vi "1D Str to ITX Wave.vi"(1 "String":string[](array[string]), 2 "Wavename":string) -> (0 "ITX Wave":string)   [LabVIEW 2020, in "Data.ITX.lvclass"]
uses:
  Data.ITX.lvclass
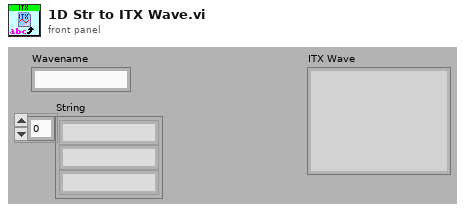
[diagram p1: front panel]
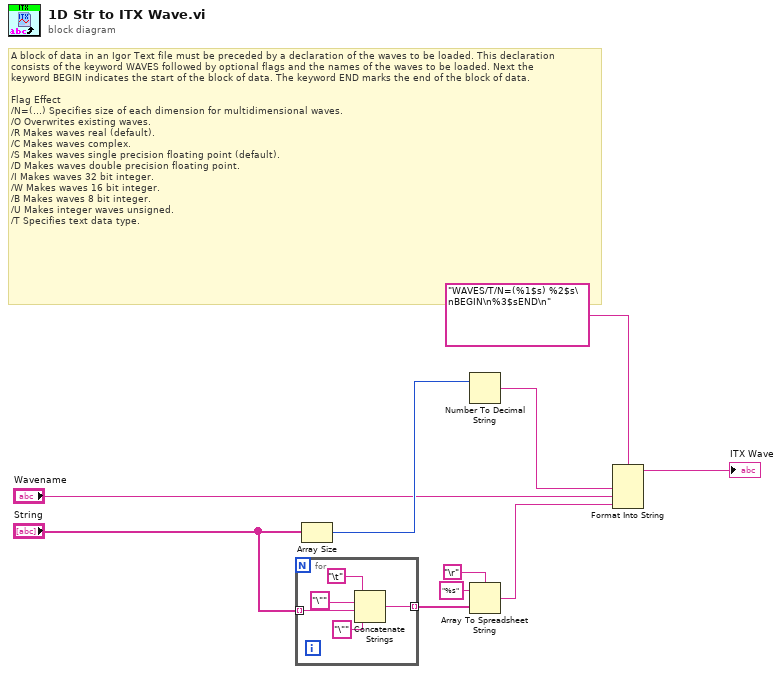
[diagram p0: block diagram]
diagram:
  # "A block of data in an Igor Text file must be preceded by a declaration of the waves to be loaded. This declaration\nconsists of the keyword WAVES followed by optional flags and the names of the waves to be loaded. Next the\nkeyword BEGIN indicates the start of the block of data. The keyword END marks the end of the block of data.\n\nFlag Effect\n/N=(…) Specifies size of each dimension for multidimensional waves.\n/O Overwrites existing waves.\n/R Makes waves real (default).\n/C Makes waves complex.\n/S Makes waves single precision floating point (default).\n/D Makes waves double precision floating point.\n/I Makes waves 32 bit integer.\n/W Makes waves 16 bit integer.\n/B Makes waves 8 bit integer.\n/U Makes integer waves unsigned.\n/T Specifies text data type."
  n1 = for {
    tunnel: "String" -> [w15] mode=indexing
    tunnel: [w14] -> w6 mode=indexing
    n2 = Concatenate Strings("\t", "\"" ("string"), w15, "\"" ("string")) -> (w14:string)
  }
  n3 = Array Size(array="String") -> (size(s)=w8:i32)
  n4 = Number To Decimal String(number=w8) -> (decimal integer string=w4:string)  [unwired: 1 out]
  n5 = Array To Spreadsheet String(delimiter (Tab)="\r", array=w6, 3:"%s" ("format string")) -> (spreadsheet string=w2:string)
  n6 = Format Into String(format string="WAVES/T/N=(%1$s) %2$s\nBEGIN\n%3$sEND\n", w4, "Wavename", w2) -> (resulting string=→"ITX Wave":string)  [unwired: 2 in, 1 out]
